vi "DB_Insert_Block.vi"(0 "Numeric (DATO)":i8=-77, 2 "date/time string":string, 5 "Numeric (DATO) 2":i8=-77, 7 "BIT (DATO)":i32=1203, 9 "BIT (DATO) 2":i32=1203, 11 "Numeric (DATO) 3":i8=-77) -> ()   [LabVIEW 2017]
uses:
  <vilib>/addons/database/Connection.llb/DB Tools Open Connec (String).vi
  <vilib>/addons/database/NI_Database_API.lvlib
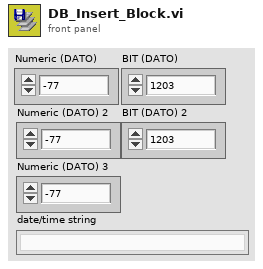
[diagram p1: front panel]
types:
  T1 = typedef "NI_Database_API.lvlib/Conn ObjectReference.ctl" = refnum<k1>
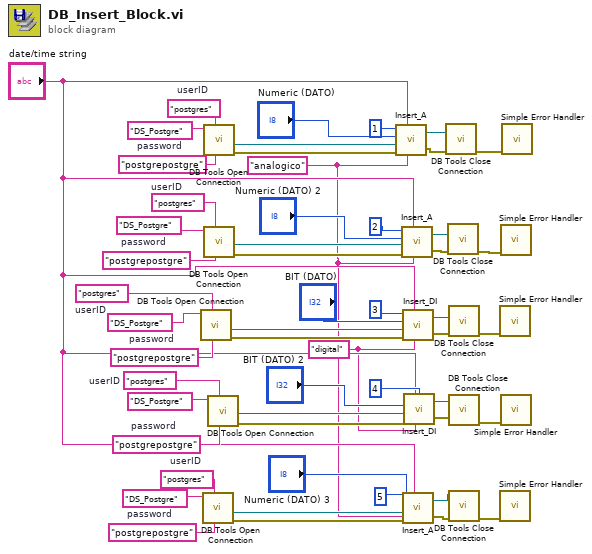
[diagram p0: block diagram]
diagram:
  w1 = "digital" ("table")
  w2 = "analogico" ("table")
  w9 = "postgrepostgre"  # password
  w11 = "postgres"  # userID
  w16 = "postgrepostgre"  # password
  w18 = "postgres"  # userID
  w23 = "postgrepostgre"  # password
  w25 = "postgres"  # userID
  w26 = "postgrepostgre"  # password
  w28 = "postgres"  # userID
  w31 = "postgrepostgre"  # password
  w33 = "postgres"  # userID
  n1 = call-poly <vilib>:"DB Tools Open Connection.vi"("password"=w9, "userID"=w11, "connection information"="DS_Postgre") -> ("error out"=w6:errorcluster, "connection reference"=w7:T1)  [unwired: 5 in]
  n2 = call-poly <vilib>:"DB Tools Open Connection.vi"("password"=w26, "userID"=w28, "connection information"="DS_Postgre") -> ("error out"=w21:errorcluster, "connection reference"=w22:T1)  [unwired: 5 in]
  n3 = call-poly <vilib>:"DB Tools Open Connection.vi"("password"=w31, "userID"=w33, "connection information"="DS_Postgre") -> ("error out"=w30:errorcluster, "connection reference"=w29:T1)  [unwired: 5 in]
  n4 = call-poly <vilib>:"DB Tools Open Connection.vi"("password"=w16, "userID"=w18, "connection information"="DS_Postgre") -> ("error out"=w15:errorcluster, "connection reference"=w14:T1)  [unwired: 5 in]
  n5 = call-poly <vilib>:"DB Tools Open Connection.vi"("password"=w23, "userID"=w25, "connection information"="DS_Postgre") -> ("error out"=w19:errorcluster, "connection reference"=w20:T1)  [unwired: 5 in]
  n6 = call "Insert_A.vi"("table"=w2, "date/time string"="date/time string", "error in (no error)"=w30, "connection reference"=w29, "Numeric (DATO)"="Numeric (DATO)", "Numeric (ID_SENSOR)"=1) -> ("error out"=w44:errorcluster, "connection reference out"=w45:T1)
  n7 = call "Insert_A.vi"("table"=w2, "date/time string"="date/time string", "error in (no error)"=w15, "connection reference"=w14, "Numeric (DATO)"="Numeric (DATO) 2", "Numeric (ID_SENSOR)"=2) -> ("error out"=w40:errorcluster, "connection reference out"=w41:T1)
  n8 = call "Insert_DI.vi"("table"=w1, "date/time string"="date/time string", "error in (no error)"=w6, "connection reference"=w7, "BIT (DATO)"="BIT (DATO)", "Numeric (ID_SENSOR)"=3) -> ("error out"=w38:errorcluster, "connection reference out"=w39:T1)
  n9 = call "Insert_A.vi"("table"=w2, "date/time string"="date/time string", "error in (no error)"=w21, "connection reference"=w22, "Numeric (DATO)"="Numeric (DATO) 3", "Numeric (ID_SENSOR)"=5) -> ("error out"=w34:errorcluster, "connection reference out"=w35:T1)
  n10 = call "Insert_DI.vi"("table"=w1, "date/time string"="date/time string", "error in (no error)"=w19, "connection reference"=w20, "BIT (DATO)"="BIT (DATO) 2", "Numeric (ID_SENSOR)"=4) -> ("error out"=w36:errorcluster, "connection reference out"=w37:T1)
  n11 = call <vilib>:"DB Tools Close Connection.vi"("error in (no error)"=w44, "connection reference"=w45) -> ("error out"=w48:errorcluster)  [unwired: 5 in]
  n12 = call <vilib>:"DB Tools Close Connection.vi"("error in (no error)"=w40, "connection reference"=w41) -> ("error out"=w47:errorcluster)  [unwired: 5 in]
  n13 = call <vilib>:"DB Tools Close Connection.vi"("error in (no error)"=w38, "connection reference"=w39) -> ("error out"=w46:errorcluster)  [unwired: 5 in]
  n14 = call <vilib>:"DB Tools Close Connection.vi"("error in (no error)"=w36, "connection reference"=w37) -> ("error out"=w43:errorcluster)  [unwired: 5 in]
  n15 = call <vilib>:"DB Tools Close Connection.vi"("error in (no error)"=w34, "connection reference"=w35) -> ("error out"=w42:errorcluster)  [unwired: 5 in]
  n16 = call <vilib>:"Simple Error Handler.vi"("error in (no error)"=w46) -> ()  [unwired: 4 in, 5 out]
  n17 = call <vilib>:"Simple Error Handler.vi"("error in (no error)"=w42) -> ()  [unwired: 4 in, 5 out]
  n18 = call <vilib>:"Simple Error Handler.vi"("error in (no error)"=w47) -> ()  [unwired: 4 in, 5 out]
  n19 = call <vilib>:"Simple Error Handler.vi"("error in (no error)"=w43) -> ()  [unwired: 4 in, 5 out]
  n20 = call <vilib>:"Simple Error Handler.vi"("error in (no error)"=w48) -> ()  [unwired: 4 in, 5 out]
